vi "TBM TOP.vi"(6 "Match Offset":cluster{"X":sgl, "Y":sgl}, 8 "Minimum Match Score":sgl=800.0, 9 "controller in":refnum<k24>, 10 "Template":path, 11 "T/B/L/R":i32) -> (0 "error out":errorcluster, 1 "Number of Matches":i32, 3 "Match(es) Found":bool)   [LabVIEW 2011]
uses:
  C:/Users/Admin/Desktop/Gantry Code Transfer/source/Code Transfer/Aerotech.A3200.dll
  Aerotech.A3200.dll
  Template change for pattern match.vi
  <vilib>/vision/driver/NI_Vision_Acquisition_Software.lvlib
  <vilib>/vision/NI_Vision_Development_Module.lvlib
panel:
  in  "Scale Factor":sgl=0.000429
  out "y rel move":dbl
  out "x rel move":dbl
  out "y":sgl
  out "x":sgl
  out "Image Out":T1(plugin-control)
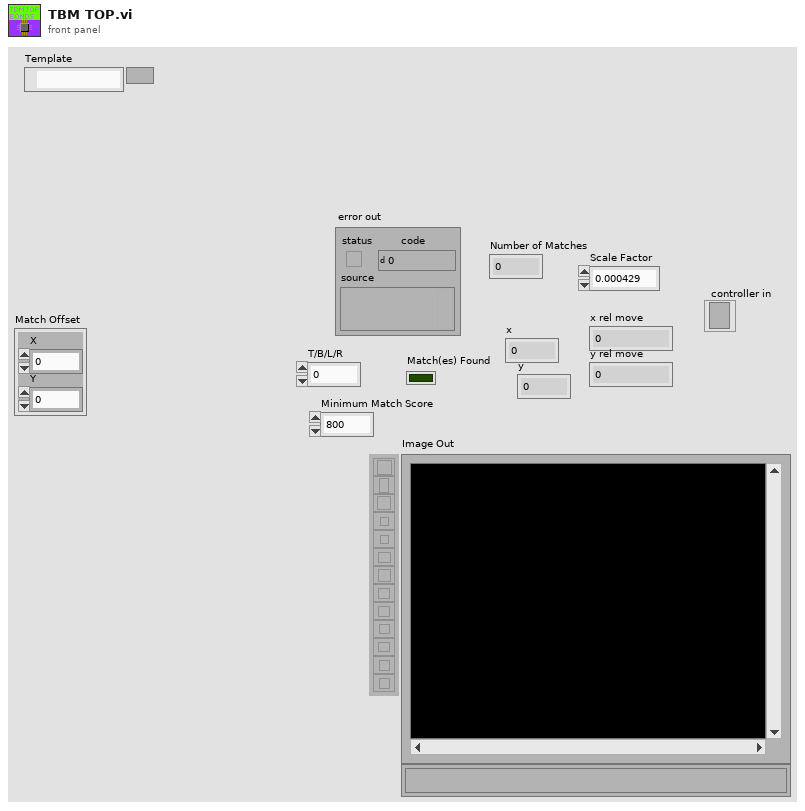
[diagram p1: front panel]
types:
  T1 = typedef "IMAQ Image.ctl" = refnum<image>
  T2 = cluster{"Global Rectangle":i32[], "Contours":cluster{"ID":enum32{"External", "Internal"}, "Type":u32, "Coordinates":i32[]}[]}
  T3 = typedef "IMAQdx.ctl" = refnum<k21>
  T4 = cluster{"Match Mode":u16, "Subpixel Accuracy":bool, "Rotation Angle Ranges (degrees)":cluster{sgl, sgl}[]}
  T5 = cluster{"Global Rectangle":i32[], "Number of Matches Requested":i32, "Minimum Match Score":sgl}
  T6 = cluster{"Position":cluster{"x":sgl, "y":sgl}, "Angle":sgl, "Scale":sgl, "Score":sgl, "Bounding Box":cluster{"x":sgl, "y":sgl}[]}[]
  T7 = cluster{"Position":cluster{"x":sgl, "y":sgl}, "Angle":sgl, "Scale":sgl, "Score":sgl, "Bounding Box":cluster{"x":sgl, "y":sgl}[]}
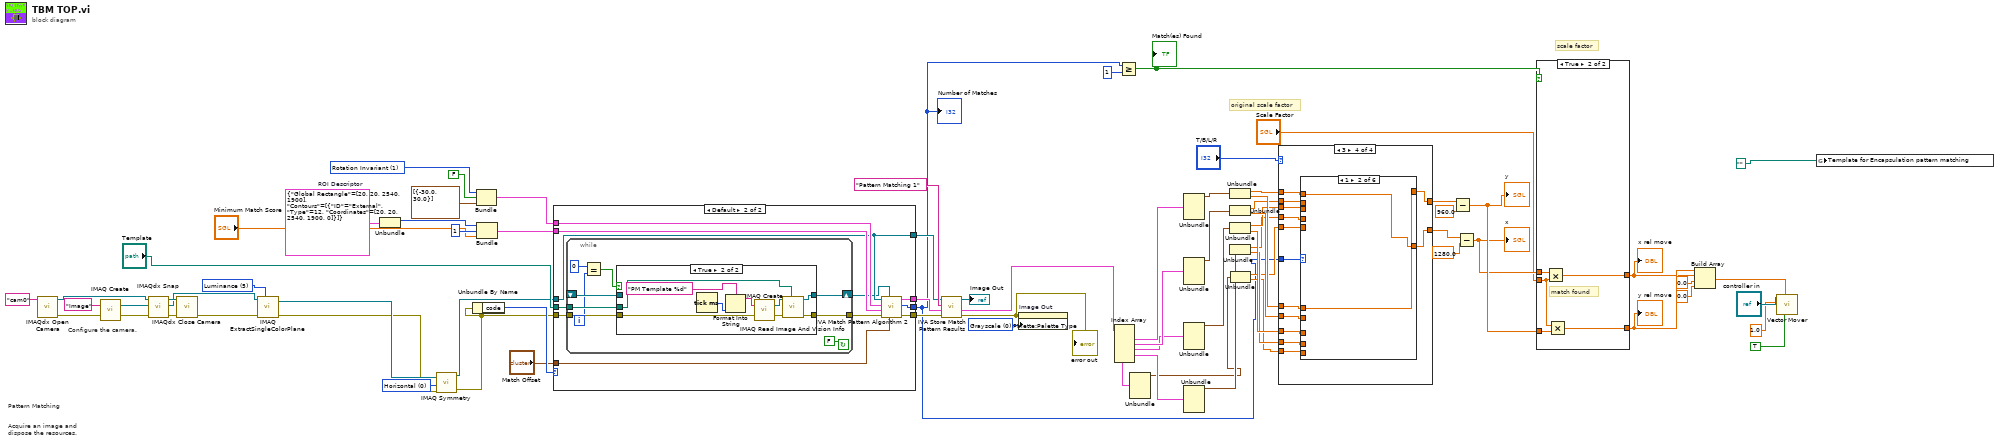
[diagram p0: block diagram]
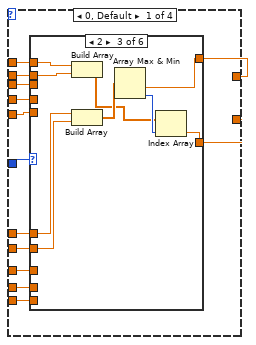
[diagram p2: hidden frame]
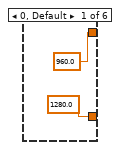
[diagram p3: hidden frame]
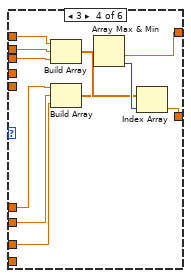
[diagram p5: hidden frame]
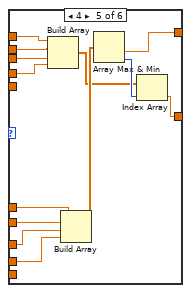
[diagram p6: hidden frame]
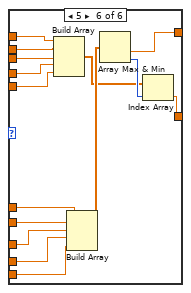
[diagram p7: hidden frame]
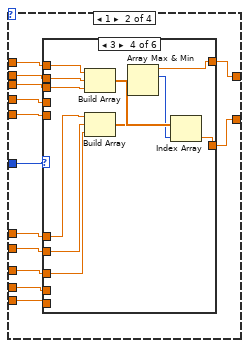
[diagram p8: hidden frame]
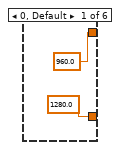
[diagram p9: hidden frame]
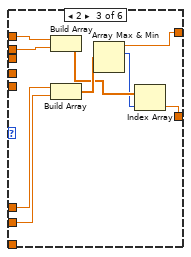
[diagram p11: hidden frame]
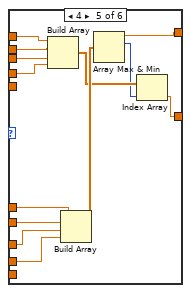
[diagram p12: hidden frame]
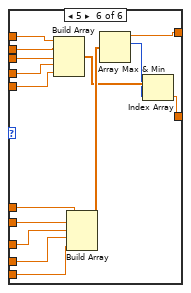
[diagram p13: hidden frame]
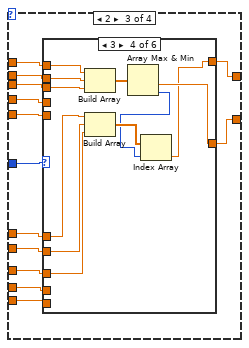
[diagram p14: hidden frame]
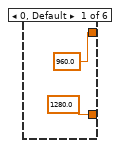
[diagram p15: hidden frame]
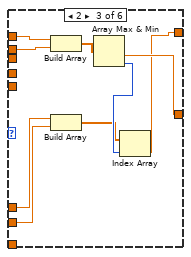
[diagram p17: hidden frame]
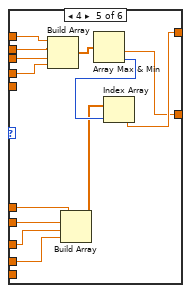
[diagram p18: hidden frame]
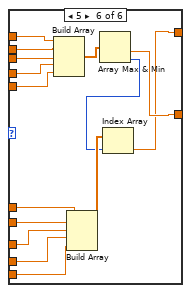
[diagram p19: hidden frame]
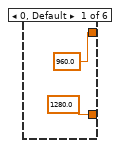
[diagram p20: hidden frame]
diagram:
  w5 = u32 0 items=["Horizontal", "Vertical", "Central", "1st Diagonal", "2nd Diagonal"] ("Type of Symmetry")
  w50 = u32 0 items=["Grayscale", "Binary", "Gradient", "Rainbow", "Temperature", "User Defined"] ("Palette")
  w65 = u16 1 items=["Shift Invariant", "Rotation Invariant"] ("Match Mode")
  w56 = T2 {"Global Rectangle"=[20, 20, 2540, 1900], "Contours"=[{"ID"=enum."External", "Type"=12, "Coordinates"=[20, 20, 2540, 1900, 0]}]}  # ROI Descriptor
  w67 = 5 items=["Red", "Green", "Blue", "Hue", "Saturation", "Luminance", "Value", "Intensity"] ("Color Plane")
  # "original scale factor"
  # "scale factor"
  # "Pattern Matching"
  # "Acquire an image and\ndispose the resources."
  # "Configure the camera."
  n1 = call <vilib>:"IMAQdx Open Camera.vi"("Session In"="cam0" ("Interface Name")) -> ("error out"=w74:errorcluster, "Session Out"=w68:T3)  [unwired: 9 in]
  n2 = call "IMAQ Create"("Image Name"="Image", "error in (no error)"=w74) -> ("New Image"=w70:T1, "error out"=w69:errorcluster)  [unwired: 3 in]
  n3 = call <vilib>:"IMAQdx Snap.vi"("error in"=w69, "Image In"=w70, "Session In"=w68) -> ("error out"=w72:errorcluster, "Image Out"=w66:T1, "Session Out"=w73:T3)  [unwired: 6 in]
  n4 = call <vilib>:"IMAQdx Close Camera.vi"("error in"=w72, "Session In"=w73) -> ("error out"=w71:errorcluster)  [unwired: 9 in]
  n5 = call "IMAQ ExtractSingleColorPlane"("Color Plane"=w67, "error in (no error)"=w71, "Image Src"=w66) -> ("error out"=w3:errorcluster, "Image Dst Out"=w4:T1)  [unwired: 7 in]
  n6 = Unbundle(w56) -> ("Global Rectangle"=w55:i32[])  [unwired: 1 out]
  n7 = call "IMAQ Symmetry"("error in (no error)"=w3, "Type of Symmetry"=w5, "Image Src"=w4) -> ("error out"=w1:errorcluster, "Image Dst Out"=w2:T1)  [unwired: 2 in]
  n8 = Unbundle By Name(w1) -> ("code"=w52:i32)
  n9 = Bundle("Match Mode"=w65, "Subpixel Accuracy"=FALSE, "Rotation Angle Ranges (degrees)"=cluster{sgl, sgl}[] [{-30.0, 30.0}]) -> (w62:T4)  [unwired: 1 in]
  n10 = Bundle "Bundle"("Global Rectangle"=w55, "Number of Matches Requested"=1, "Minimum Match Score"="Minimum Match Score") -> (w59:T5)  [unwired: 1 in]
  n11 = case shown="Default" w52 {
    tunnel: "Template" -> [_ w81]
    tunnel: w1 -> [_ w80]
    tunnel: [_ w88] -> w9
    tunnel: w62 -> [_ w87]
    tunnel: w59 -> [_ w86]
    tunnel: "Match Offset" -> [_ w85]
    tunnel: w2 -> [w77 w82]
    tunnel: [_ w84] -> w57
    tunnel: [_ w83] -> w54
    tunnel: [w77 w82] -> w53
    frame -1074396199, -1074396198 {
      # "Discard\nCoordinate\nSystem Error"
    }
    frame Default {
      n12 = while {
        shift-right: [w97] -> w78
        shift-left: _ -> [w96]
        tunnel: [w94] -> w79
        tunnel: w80 -> [w93]
        tunnel: w81 -> [w92]
        i -> [w91]
        stop <- FALSE continue-if-true
        n13 = Equal?(x=0, y=w91) -> (x = y?=w89:bool)
        n14 = case shown="True" w89 {
          tunnel: [w99 w105] -> w97
          tunnel: w96 -> [w99 _]
          tunnel: [w98 w102] -> w94
          tunnel: w93 -> [w98 w101]
          tunnel: w92 -> [_ w100]
          frame False {
          }
          frame True {
            n15 = Tick Count (ms)() -> (millisecond timer value=w108:u32)
            n16 = Format Into String(format string="PM Template %d" ("Image Name"), w108) -> (resulting string=w107:string)  [unwired: 2 in, 1 out]
            n17 = call "IMAQ Create"("Image Name"=w107, "error in (no error)"=w101) -> ("New Image"=w104:T1, "error out"=w103:errorcluster)  [unwired: 3 in]
            n18 = call "IMAQ Read Image And Vision Info"("File Path"=w100, "error in (no error)"=w103, "Image"=w104) -> ("error out"=w102:errorcluster, "Image Out"=w105:T1)  [unwired: 6 in, 1 out]
          }
        }
      }
      n19 = call <vilib>:"IVA Match Pattern Algorithm 2.vi"("Match Offset"=w85, "Image Template"=w78, "error in (no error)"=w79, "Match Parameters"=w86, "Setup Match Parameters"=w87, "Image"=w82) -> ("error out"=w84:errorcluster, "Number of Matches"=w88:i32, "Matches"=w83:T6)  [unwired: 3 in]
    }
  }
  "Number of Matches" <- w9
  n20 = call <vilib>:"IVA Store Match Pattern Results.vi"("error in (no error)"=w57, "Matches"=w54, "Step Name"="Pattern Matching 1", "Image in"=w53) -> ("error out"=w10:errorcluster, "Calibrated Matches"=w11:T6, "Image dup"=→"Image Out":T1)  [unwired: 5 in]
  "error out" <- w10
  n21 = property on="Image Out" class="ImageControl"(error in=w10, "Palette:Palette Type"=w50) -> ()  [unwired: 1 in, 2 out]
  n22 = Index Array(array=w11) -> (element #1=w46:T7, element #2=w45:T7, element #3=w44:T7, element #4=w43:T7, element #5=w23:T7)  [unwired: 5 in]
  n23 = Greater Or Equal?(x=w9, y=1) -> (x >= y?=w36:bool)
  "Match(es) Found" <- w36
  n24 = Unbundle(w23) -> ("Position"=w22:cluster{"x":sgl, "y":sgl})  [unwired: 4 out]
  n25 = Unbundle(w46) -> ("Position"=w39:cluster{"x":sgl, "y":sgl})  [unwired: 4 out]
  n26 = Unbundle(w45) -> ("Position"=w40:cluster{"x":sgl, "y":sgl})  [unwired: 4 out]
  n27 = Unbundle(w44) -> ("Position"=w41:cluster{"x":sgl, "y":sgl})  [unwired: 4 out]
  n28 = Unbundle(w43) -> ("Position"=w42:cluster{"x":sgl, "y":sgl})  [unwired: 4 out]
  n29 = Unbundle(w39) -> ("x"=w33:sgl, "y"=w32:sgl)
  n30 = Unbundle(w40) -> ("x"=w31:sgl, "y"=w30:sgl)
  n31 = Unbundle(w41) -> ("x"=w28:sgl, "y"=w27:sgl)
  n32 = Unbundle(w42) -> ("x"=w24:sgl, "y"=w26:sgl)
  n33 = Unbundle(w22) -> ("x"=w21:sgl, "y"=w20:sgl)
  n34 = case shown="3" "T/B/L/R" {
    tunnel: w33 -> [w121 w186 w251 w316]
    tunnel: w32 -> [w120 w181 w246 w311]
    tunnel: w31 -> [w119 w185 w250 w315]
    tunnel: w30 -> [w118 w180 w245 w310]
    tunnel: [w117 w175 w240 w305] -> w29
    tunnel: w28 -> [w116 w184 w249 w314]
    tunnel: w27 -> [w115 w179 w244 w309]
    tunnel: w26 -> [w114 w178 w243 w308]
    tunnel: [w113 w176 w241 w306] -> w25
    tunnel: w24 -> [w112 w183 w248 w313]
    tunnel: w21 -> [w111 w182 w247 w312]
    tunnel: w20 -> [w110 w177 w242 w307]
    tunnel: w9 -> [w109 w174 w239 w304]
    frame 0, Default {
      n35 = case shown="2" w109 {
        tunnel: w121 -> [_ w124 w134 w142 w155 w170]
        tunnel: w120 -> [_ w125 w132 w139 w151 w166]
        tunnel: [sgl 960.0 ("y") w125 w129 w144 w157 w172] -> w117
        tunnel: w119 -> [_ _ w133 w141 w154 w169]
        tunnel: w118 -> [_ _ w131 w138 w150 w165]
        tunnel: w116 -> [_ _ _ w140 w153 w168]
        tunnel: w115 -> [_ _ _ w137 w149 w164]
        tunnel: w114 -> [_ _ _ _ w148 w163]
        tunnel: [sgl 1280.0 ("x") w124 w126 w143 w156 w171] -> w113
        tunnel: w112 -> [_ _ _ _ w152 w167]
        tunnel: w111 -> [_ _ _ _ _ w160]
        tunnel: w110 -> [_ _ _ _ _ w159]
        frame 0, Default {
        }
        frame 1 {
        }
        frame 2 {
          n36 = Build Array(w134, w133) -> (w127:sgl[])
          n37 = Build Array(w132, w131) -> (w128:sgl[])
          n38 = Array Max & Min(array=w128) -> (min value=w129:sgl, min index (indices)=w130:i32)  [unwired: 2 out]
          n39 = Index Array(array=w127, index=w130) -> (element=w126:sgl)
        }
        frame 3 {
          n40 = Build Array(w142, w141, w140) -> (w136:sgl[])
          n41 = Build Array(w139, w138, w137) -> (w135:sgl[])
          n42 = Array Max & Min(array=w135) -> (min value=w144:sgl, min index (indices)=w145:i32)  [unwired: 2 out]
          n43 = Index Array(array=w136, index=w145) -> (element=w143:sgl)
        }
        frame 4 {
          n44 = Build Array(w155, w154, w153, w152) -> (w146:sgl[])
          n45 = Build Array(w151, w150, w149, w148) -> (w147:sgl[])
          n46 = Array Max & Min(array=w147) -> (min value=w157:sgl, min index (indices)=w158:i32)  [unwired: 2 out]
          n47 = Index Array(array=w146, index=w158) -> (element=w156:sgl)
        }
        frame 5 {
          n48 = Build Array(w170, w169, w168, w167, w160) -> (w161:sgl[])
          n49 = Build Array(w166, w165, w164, w163, w159) -> (w162:sgl[])
          n50 = Array Max & Min(array=w162) -> (min value=w172:sgl, min index (indices)=w173:i32)  [unwired: 2 out]
          n51 = Index Array(array=w161, index=w173) -> (element=w171:sgl)
        }
      }
    }
    frame 1 {
      n52 = case shown="3" w174 {
        tunnel: w186 -> [_ w189 w199 w209 w222 w237]
        tunnel: w181 -> [_ w190 w197 w206 w218 w233]
        tunnel: [sgl 960.0 ("y") w190 w192 w201 w212 w225] -> w175
        tunnel: w185 -> [_ _ w198 w208 w221 w236]
        tunnel: w180 -> [_ _ w196 w205 w217 w232]
        tunnel: w184 -> [_ _ _ w207 w220 w235]
        tunnel: w179 -> [_ _ _ w204 w216 w231]
        tunnel: w178 -> [_ _ _ _ w215 w230]
        tunnel: [sgl 1280.0 ("x") w189 w193 w210 w223 w238] -> w176
        tunnel: w183 -> [_ _ _ _ w219 w234]
        tunnel: w182 -> [_ _ _ _ _ w227]
        tunnel: w177 -> [_ _ _ _ _ w226]
        frame 0, Default {
        }
        frame 1 {
        }
        frame 2 {
          n53 = Build Array(w199, w198) -> (w194:sgl[])
          n54 = Build Array(w197, w196) -> (w195:sgl[])
          n55 = Array Max & Min(array=w195) -> (max value=w192:sgl, max index (indices)=w191:i32)  [unwired: 2 out]
          n56 = Index Array(array=w194, index=w191) -> (element=w193:sgl)
        }
        frame 3 {
          n57 = Build Array(w209, w208, w207) -> (w203:sgl[])
          n58 = Build Array(w206, w205, w204) -> (w202:sgl[])
          n59 = Array Max & Min(array=w202) -> (max value=w201:sgl, max index (indices)=w200:i32)  [unwired: 2 out]
          n60 = Index Array(array=w203, index=w200) -> (element=w210:sgl)
        }
        frame 4 {
          n61 = Build Array(w222, w221, w220, w219) -> (w213:sgl[])
          n62 = Build Array(w218, w217, w216, w215) -> (w214:sgl[])
          n63 = Array Max & Min(array=w214) -> (max value=w212:sgl, max index (indices)=w211:i32)  [unwired: 2 out]
          n64 = Index Array(array=w213, index=w211) -> (element=w223:sgl)
        }
        frame 5 {
          n65 = Build Array(w237, w236, w235, w234, w227) -> (w228:sgl[])
          n66 = Build Array(w233, w232, w231, w230, w226) -> (w229:sgl[])
          n67 = Array Max & Min(array=w229) -> (max value=w225:sgl, max index (indices)=w224:i32)  [unwired: 2 out]
          n68 = Index Array(array=w228, index=w224) -> (element=w238:sgl)
        }
      }
    }
    frame 2 {
      n69 = case shown="3" w239 {
        tunnel: w251 -> [_ w254 w264 w275 w287 w303]
        tunnel: w246 -> [_ w255 w262 w272 w283 w299]
        tunnel: [sgl 960.0 ("y") w255 w256 w265 w277 w289] -> w240
        tunnel: w250 -> [_ _ w263 w274 w286 w302]
        tunnel: w245 -> [_ _ w261 w271 w282 w298]
        tunnel: w249 -> [_ _ _ w273 w285 w301]
        tunnel: w244 -> [_ _ _ w270 w281 w297]
        tunnel: w243 -> [_ _ _ _ w280 w296]
        tunnel: [sgl 1280.0 ("x") w254 w259 w266 w276 w290] -> w241
        tunnel: w248 -> [_ _ _ _ w284 w300]
        tunnel: w247 -> [_ _ _ _ _ w295]
        tunnel: w242 -> [_ _ _ _ _ w294]
        frame 0, Default {
        }
        frame 1 {
        }
        frame 2 {
          n70 = Build Array(w264, w263) -> (w260:sgl[])
          n71 = Build Array(w262, w261) -> (w257:sgl[])
          n72 = Array Max & Min(array=w260) -> (min value=w259:sgl, min index (indices)=w258:i32)  [unwired: 2 out]
          n73 = Index Array(array=w257, index=w258) -> (element=w256:sgl)
        }
        frame 3 {
          n74 = Build Array(w275, w274, w273) -> (w269:sgl[])
          n75 = Build Array(w272, w271, w270) -> (w268:sgl[])
          n76 = Array Max & Min(array=w269) -> (min value=w266:sgl, min index (indices)=w267:i32)  [unwired: 2 out]
          n77 = Index Array(array=w268, index=w267) -> (element=w265:sgl)
        }
        frame 4 {
          n78 = Build Array(w287, w286, w285, w284) -> (w278:sgl[])
          n79 = Build Array(w283, w282, w281, w280) -> (w279:sgl[])
          n80 = Array Max & Min(array=w278) -> (min value=w276:sgl, min index (indices)=w288:i32)  [unwired: 2 out]
          n81 = Index Array(array=w279, index=w288) -> (element=w277:sgl)
        }
        frame 5 {
          n82 = Build Array(w303, w302, w301, w300, w295) -> (w291:sgl[])
          n83 = Build Array(w299, w298, w297, w296, w294) -> (w293:sgl[])
          n84 = Array Max & Min(array=w291) -> (min value=w290:sgl, min index (indices)=w292:i32)  [unwired: 2 out]
          n85 = Index Array(array=w293, index=w292) -> (element=w289:sgl)
        }
      }
    }
    frame 3 {
      n86 = case shown="1" w304 {
        tunnel: w316 -> [_ w319 w329 w340 w353 w368]
        tunnel: w311 -> [_ w320 w327 w337 w349 w364]
        tunnel: [sgl 960.0 ("y") w320 w323 w332 w343 w356] -> w305
        tunnel: w315 -> [_ _ w328 w339 w352 w367]
        tunnel: w310 -> [_ _ w326 w336 w348 w363]
        tunnel: w314 -> [_ _ _ w338 w351 w366]
        tunnel: w309 -> [_ _ _ w335 w347 w362]
        tunnel: w308 -> [_ _ _ _ w346 w361]
        tunnel: [sgl 1280.0 ("x") w319 w322 w331 w342 w355] -> w306
        tunnel: w313 -> [_ _ _ _ w350 w365]
        tunnel: w312 -> [_ _ _ _ _ w360]
        tunnel: w307 -> [_ _ _ _ _ w359]
        frame 0, Default {
        }
        frame 1 {
        }
        frame 2 {
          n87 = Build Array(w329, w328) -> (w325:sgl[])
          n88 = Build Array(w327, w326) -> (w324:sgl[])
          n89 = Array Max & Min(array=w325) -> (max value=w322:sgl, max index (indices)=w321:i32)  [unwired: 2 out]
          n90 = Index Array(array=w324, index=w321) -> (element=w323:sgl)
        }
        frame 3 {
          n91 = Build Array(w340, w339, w338) -> (w334:sgl[])
          n92 = Build Array(w337, w336, w335) -> (w333:sgl[])
          n93 = Array Max & Min(array=w334) -> (max value=w331:sgl, max index (indices)=w330:i32)  [unwired: 2 out]
          n94 = Index Array(array=w333, index=w330) -> (element=w332:sgl)
        }
        frame 4 {
          n95 = Build Array(w353, w352, w351, w350) -> (w344:sgl[])
          n96 = Build Array(w349, w348, w347, w346) -> (w345:sgl[])
          n97 = Array Max & Min(array=w344) -> (max value=w342:sgl, max index (indices)=w341:i32)  [unwired: 2 out]
          n98 = Index Array(array=w345, index=w341) -> (element=w343:sgl)
        }
        frame 5 {
          n99 = Build Array(w368, w367, w366, w365, w360) -> (w357:sgl[])
          n100 = Build Array(w364, w363, w362, w361, w359) -> (w358:sgl[])
          n101 = Array Max & Min(array=w357) -> (max value=w355:sgl, max index (indices)=w354:i32)  [unwired: 2 out]
          n102 = Index Array(array=w358, index=w354) -> (element=w356:sgl)
        }
      }
    }
  }
  n103 = Subtract(x=w29, y=sgl 960.0) -> (x-y=w49:sgl)
  "y" <- w49
  n104 = Subtract(x=w25, y=sgl 1280.0) -> (x-y=w48:sgl)
  "x" <- w48
  n105 = case shown="True" w36 {
    tunnel: w49 -> [_ w374]
    tunnel: w48 -> [_ w373]
    tunnel: [w369 w372] -> w34
    tunnel: [w369 w371] -> w35
    tunnel: "Scale Factor" -> [_ w370]
    frame False {
      w369 = sgl 0.0
      # "no match found"
    }
    frame True {
      # "match found"
      n106 = Multiply(x=w373, y=w370) -> (x*y=w372:sgl)
      n107 = Multiply(x=w370, y=w374) -> (x*y=w371:sgl)
    }
  }
  "x rel move" <- w34
  "y rel move" <- w35
  n108 = Build Array(w35, w34, 0.0 ("element"), 0.0 ("element")) -> (w12:dbl[])
  n109 = call "Vector Mover.vi"("Absolute/Relative (F/T)"=TRUE, "Movement Vector"=w12, "Vector Speed"=1.0, "controller in"="controller in") -> ()  [unwired: 2 in, 4 out]
  n110 = global write "Template change for pattern match.vi" "Template for Encapsulation pattern matching"(path "") -> ()
